vi "Read Channel Array.vi"(8 "error in":errorcluster, 10 "channels":refnum<class "Channel.lvclass">[](array[class]), 11 "digital mode in":refnum<class "Digital Mode.lvclass">) -> (0 "error out":errorcluster, 2 "channel settings":T1[](array[typedef]), 3 "digital mode out":refnum<class "Digital Mode.lvclass">)   [LabVIEW 2020, in "Scan Engine Scripting.lvlib" / "Digital Mode.lvclass"]
uses:
  Digital Mode.lvclass
  Channel Classes/Channel/Channel.lvclass
  Controls/digital channel settings.ctl
  Digital Mode.lvclass/Digital Mode.ctl
  Channel Classes/Digital Channel/Digital Channel.lvclass
  Scan Engine Scripting.lvlib
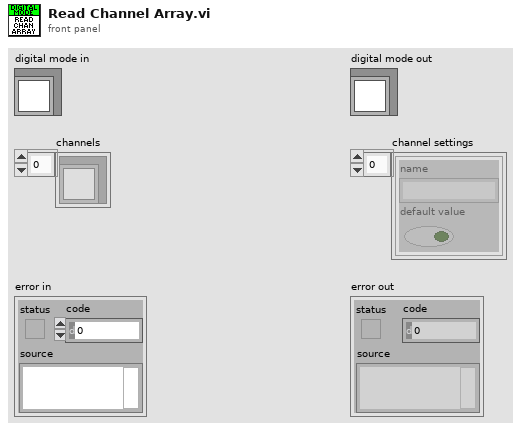
[diagram p1: front panel]
types:
  T1 = typedef "Scan Engine Scripting.lvlib/digital channel settings.ctl" = cluster{"name":string, "default value":bool}
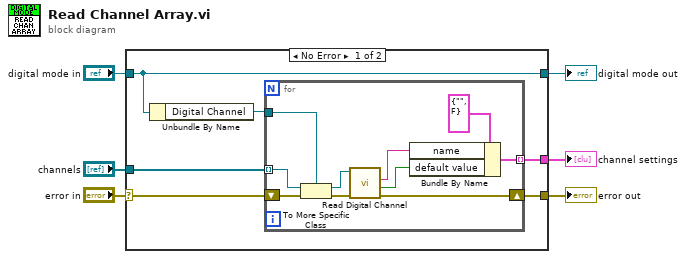
[diagram p0: block diagram]
diagram:
  n1 = case shown="No Error" "error in" {
    selector: "error in" -> [w11 w24]
    tunnel: [w10 w24] -> w5
    tunnel: [w8 w23] -> w3
    tunnel: "digital mode in" -> [w8 w23]
    tunnel: "channels" -> [w12 _]
    tunnel: [w9 _] -> w1
    frame No Error {
      n2 = Unbundle By Name(w8) -> ("Digital Channel"=w7:refnum<class "Digital Channel.lvclass">)
      n3 = for {
        tunnel: w12 -> [w19] mode=indexing
        tunnel: [w21] -> w9 mode=indexing
        shift-right: [w16] -> w10
        shift-left: w11 -> [w20]
        tunnel: w7 -> [w13]
        n4 = To More Specific Class(target class=w13, reference=w19, error in=w20) -> (specific class reference=w17:refnum<class "Digital Channel.lvclass">, error out=w18:errorcluster)
        n5 = call "Read Digital Channel.vi"("error in"=w18, "digital channel in"=w17) -> ("error out"=w16:errorcluster, "default value"=w15:bool, "name"=w14:string)  [unwired: 5 in, 2 out]
        n6 = Bundle By Name(cluster=T1 {"name"="", "default value"=FALSE} ("channel settings"), "name"=w14, "default value"=w15) -> (w21:T1)
      }
    }
    frame Error {
    }
  }
  "error out" <- w5
  "digital mode out" <- w3
  "channel settings" <- w1
